vi "graphs.vi"() -> ()   [LabVIEW 2021]
uses:
  CALIBRATION.lvlib
panel:
  in  "Tab Control":T1(tab)
  out "analog_hysteresis":T2(graph)
  out "digital_hysteresis":T3(graph)
  out "salita_confronto_grafico":T3(graph)
  out "discesa_confronto_grafico":T3(graph)
  out "graph":T3(graph)
  in  "digital_s2":path=path "C:/Users/anton/myUnisannio/magistrale/MAPI/esame/miriam_pc/last/digitale/tab_salita2.csv"
  in  "digital_s1":path=path "C:/Users/anton/myUnisannio/magistrale/MAPI/esame/miriam_pc/last/digitale/tab_salita1.csv"
  in  "digital_d2":path=path "C:/Users/anton/myUnisannio/magistrale/MAPI/esame/miriam_pc/last/digitale/tab_discesa2.csv"
  in  "digital_d1":path=path "C:/Users/anton/myUnisannio/magistrale/MAPI/esame/miriam_pc/last/digitale/tab_discesa1.csv"
  in  "analog_d2":path=path "C:/Users/anton/myUnisannio/magistrale/MAPI/esame/miriam_pc/last/analogico/tab_discesa2.csv"
  in  "analog_d1":path=path "C:/Users/anton/myUnisannio/magistrale/MAPI/esame/miriam_pc/last/analogico/tab_discesa1.csv"
  in  "analog_s2":path=path "C:/Users/anton/myUnisannio/magistrale/MAPI/esame/miriam_pc/last/analogico/tab_salita2.csv"
  in  "analog_s1":path=path "C:/Users/anton/myUnisannio/magistrale/MAPI/esame/miriam_pc/last/analogico/tab_salita1.csv"
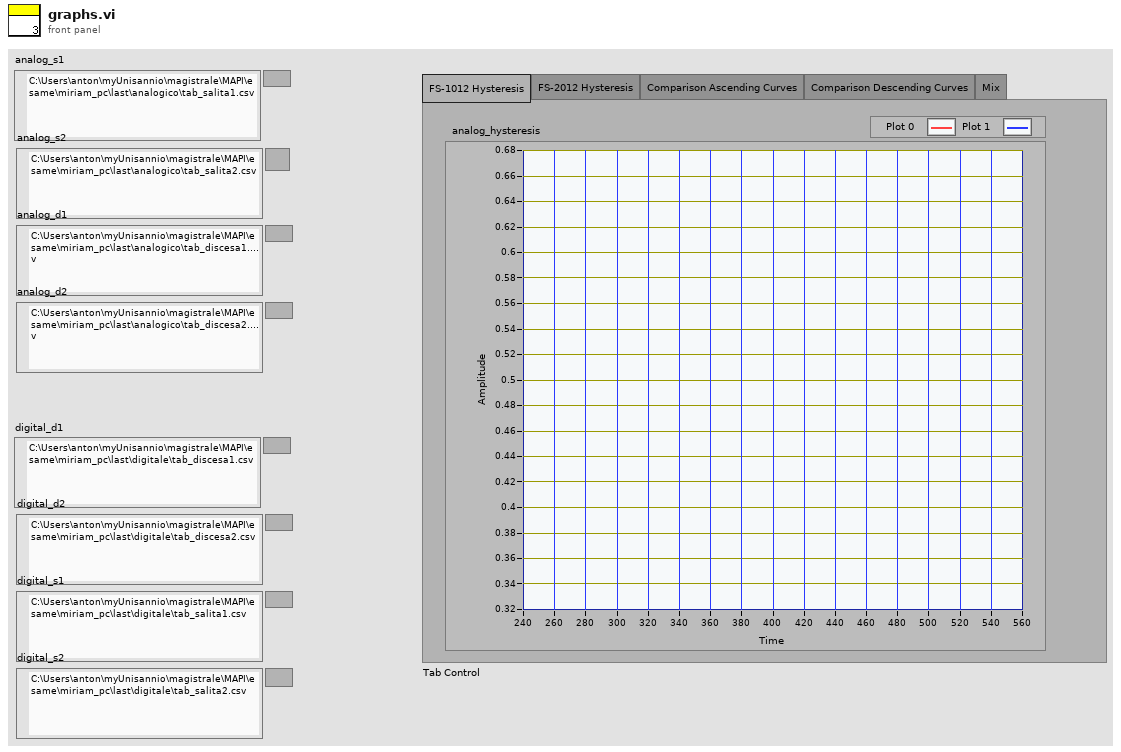
[diagram p1: front panel]
types:
  T1 = enum32{"FS-1012 Hysteresis", "FS-2012 Hysteresis", "Comparison Ascending Curves", "Comparison Descending Curves", "Mix"}
  T2 = cluster{"analog_s":dbl[], "current_values":dbl[]}[]
  T3 = cluster{"current_values":dbl[], "digital_d":dbl[]}[]
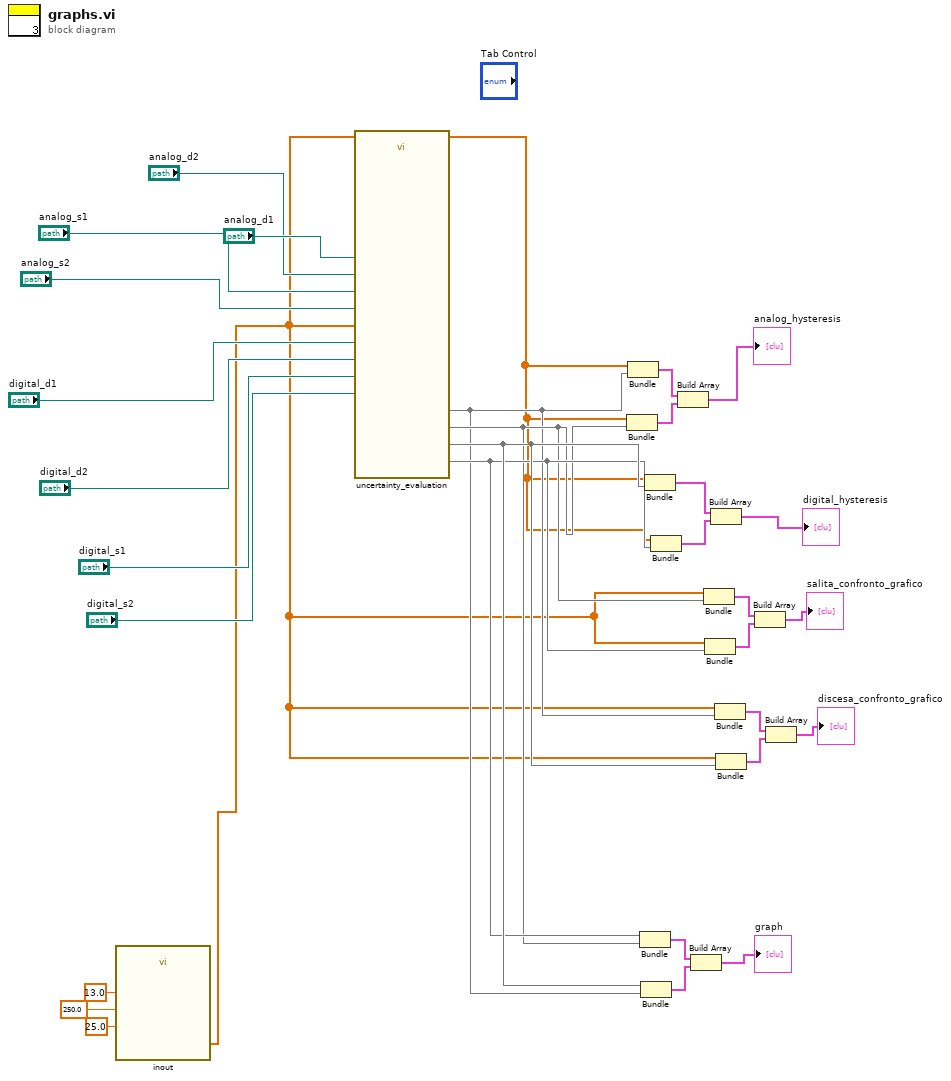
[diagram p0: block diagram]
diagram:
  n1 = call "inout.vi"("Step [mA]"=25.0, "Initial Value [mA]"=250.0, "# Steps"=13.0) -> ("Array"=w4:dbl[])  [unwired: 8 in]
  n2 = call "uncertainty_evaluation.vi"(0:"analog_s1", 2:"analog_s2", 3:w4, 5:"digital_s1", 6:"digital_s2", 10:"analog_d1", 11:"digital_d1", 12:"analog_d2", 13:"digital_d2") -> (19:w8, 21:w5, 24:w6, 27:w7)  [unwired: 15 in]
  n3 = Bundle("Array"=w4, w6) -> (w23:cluster{"Array":dbl[], void})  [unwired: 1 in]
  n4 = Bundle("Array"=w4, w5) -> (w22:cluster{"Array":dbl[], void})  [unwired: 1 in]
  n5 = Bundle(w7, w6) -> (w11:cluster{void, void})  [unwired: 1 in]
  n6 = Bundle(w8, w5) -> (w10:cluster{void, void})  [unwired: 1 in]
  n7 = Bundle("Array"=w4, w8) -> (w20:cluster{"Array":dbl[], void})  [unwired: 1 in]
  n8 = Bundle("Array"=w4, w7) -> (w19:cluster{"Array":dbl[], void})  [unwired: 1 in]
  n9 = Build Array(w22, w23) -> (→"analog_hysteresis":cluster{"Array":dbl[], void}[])
  n10 = Build Array(w11, w10) -> (→"graph":cluster{void, void}[])
  n11 = Bundle("Array"=w4, w6) -> (w17:cluster{"Array":dbl[], void})  [unwired: 1 in]
  n12 = Bundle("Array"=w4, w7) -> (w16:cluster{"Array":dbl[], void})  [unwired: 1 in]
  n13 = Build Array(w20, w19) -> (→"digital_hysteresis":cluster{"Array":dbl[], void}[])
  n14 = Bundle("Array"=w4, w5) -> (w12:cluster{"Array":dbl[], void})  [unwired: 1 in]
  n15 = Bundle("Array"=w4, w8) -> (w13:cluster{"Array":dbl[], void})  [unwired: 1 in]
  n16 = Build Array(w17, w16) -> (→"salita_confronto_grafico":cluster{"Array":dbl[], void}[])
  n17 = Build Array(w12, w13) -> (→"discesa_confronto_grafico":cluster{"Array":dbl[], void}[])
